vi "Test-CryptoNight-Step-3.vi"() -> ()   [LabVIEW 2017]
panel:
  out "Values Match?":bool
  out "exp_hp_state_out":u8[](array[numeric]) format="%.0x"
  out "Runtime (minutes)":dbl
  in  "Override Iterations":bool=TRUE
  out "Runtime (s)":dbl
  out "Runtime (ms)":u32
  in  "# of Iterations":i32
  out "hp_state out":u8[](array[numeric]) format="%.0x"
  out "b_out":u64[](array[numeric]) format="%.0x"
  out "a_out":u64[](array[numeric]) format="%.0x"
  in  "FileName":string="log_file.8.bin"
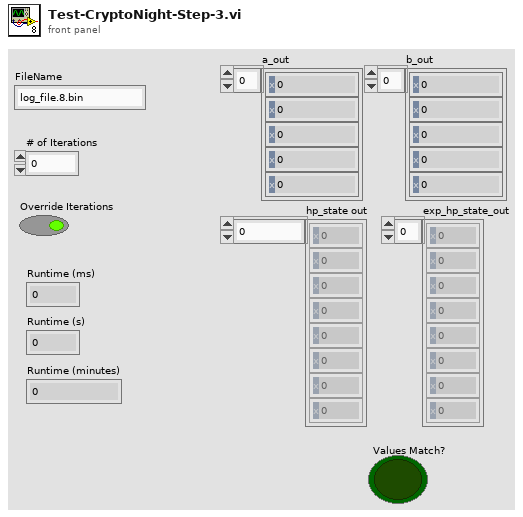
[diagram p1: front panel]
types:
  T1 = cluster{"a":u64[], "b":u64[], "hp_state_in":u8[], "hp_state_out":u8[]}
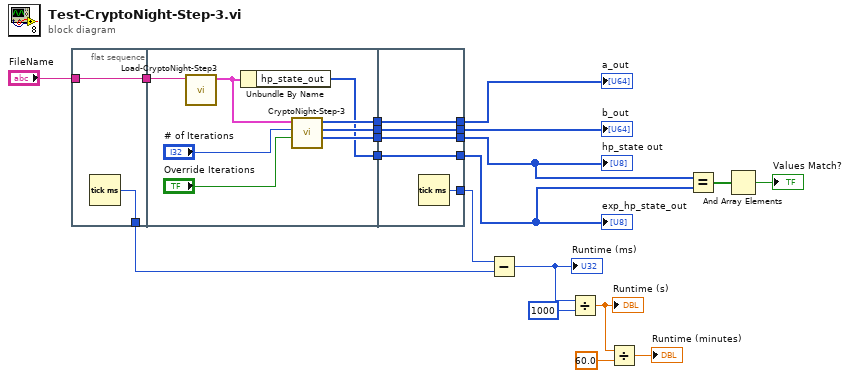
[diagram p0: block diagram]
diagram:
  n1 = flat-sequence {
    tunnel: "FileName" -> [w21]
    tunnel: [w21] -> w13
    tunnel: [w20] -> w11
    tunnel: [w29] -> w16
    tunnel: [w28] -> w15
    tunnel: [w27] -> w14
    tunnel: w13 -> [w24]
    tunnel: [w22] -> w5
    tunnel: [w32] -> w4
    tunnel: [w33] -> w17
    tunnel: [w34] -> w18
    tunnel: w16 -> [w34]
    tunnel: w15 -> [w33]
    tunnel: w14 -> [w32]
    tunnel: [w31] -> w12
    tunnel: [w30] -> w3
    tunnel: w5 -> [w30]
    frame #0 {
      n2 = Tick Count (ms)() -> (millisecond timer value=w20:u32)
    }
    frame #1 {
      n3 = call "Load-CryptoNight-Step3.vi"("FileName"=w24) -> ("output cluster"=w23:T1)  [unwired: 9 in, 1 out]
      n4 = Unbundle By Name(w23) -> ("hp_state_out"=w22:u8[])
      n5 = call "CryptoNight-Step-3.vi"("Override Iterations"="Override Iterations", "# of Iterations"="# of Iterations", "input cluster"=w23) -> ("hp_state out"=w27:u8[], "b_out"=w28:u64[], "a_out"=w29:u64[])  [unwired: 6 in]
    }
    frame #2 {
      n6 = Tick Count (ms)() -> (millisecond timer value=w31:u32)
    }
  }
  n7 = Subtract(x=w12, y=w11) -> (x-y=w10:u32)
  "Runtime (ms)" <- w10
  n8 = Divide(x=w10, y=u32 1000) -> (x/y=w8:dbl)
  "Runtime (s)" <- w8
  n9 = Divide(x=w8, y=60.0) -> (x/y=→"Runtime (minutes)":dbl)
  n10 = Equal?(x=w4, y=w3) -> (x = y?=w2:bool[])
  n11 = And Array Elements(Boolean array=w2) -> (logical AND=→"Values Match?":bool)
  "a_out" <- w18
  "b_out" <- w17
  "hp_state out" <- w4
  "exp_hp_state_out" <- w3
